vi "LVClass_ModalCoef ctor.vi"(0 "ModalCoef in":refnum<class "ModalCoef.lvclass">, 5 "TypePhase":T1, 11 "error in (no error)":errorcluster) -> (4 "ModalCoef out":refnum<class "ModalCoef.lvclass">, 15 "error out":errorcluster)   [LabVIEW 2020, in "ModalCoef.lvclass"]
doc: "ModalCoef constructor.\n\n--------------------------------------------------------------------------------\n\n<B>ModalCoefIn </B> : Constant Pointer to ModalCoef object.\n<B>ModalCoefOut </B> : Constant Pointer to ModalCoef object.\n<B>TypePhase </B> : TypePhase Phase mode reconstruction.\n<B>ErrorIn </B> : Error\n<B>ErrorOut </B> : Error\n\n--------------------------------------------------------------------------------"
uses:
  ModalCoef.lvclass
  WavefrontModalReconstructionType.ctl
  Handle creation.ctl
  ModalCoef.lvclass/ModalCoef.ctl
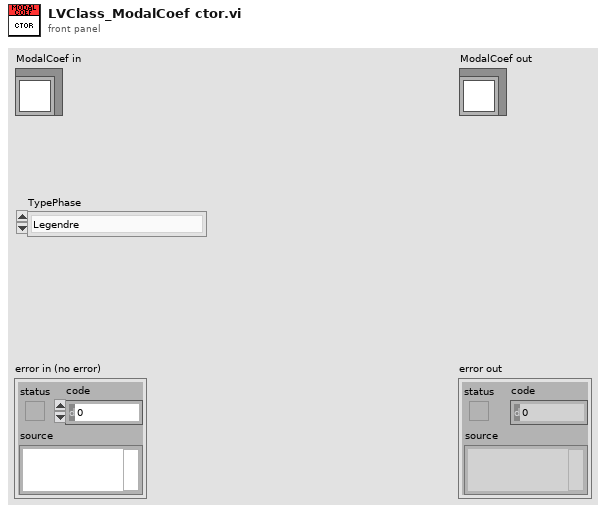
[diagram p1: front panel]
types:
  T1 = typedef "WavefrontModalReconstructionType.ctl" = enum16{"Legendre", "Zernike"}
  T2 = typedef "Handle creation.ctl" = enum16{"By ctor", "By write function"}
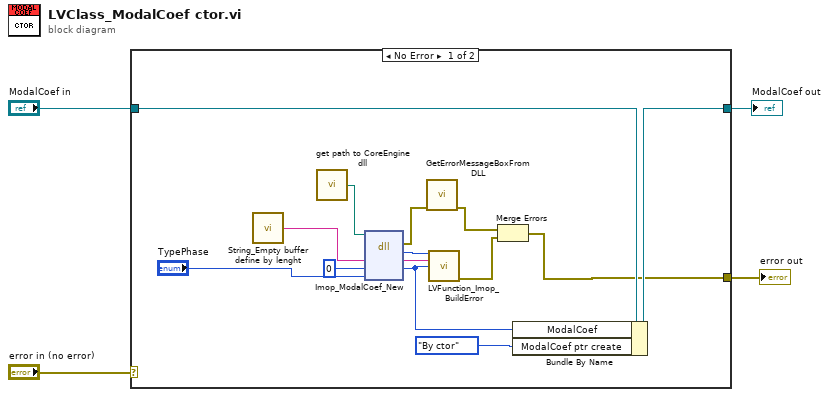
[diagram p0: block diagram]
diagram:
  n1 = case shown="No Error" "error in (no error)" {
    selector: "error in (no error)" -> [_ w20]
    tunnel: [w6 w20] -> w3
    tunnel: [w10 w19] -> w1
    tunnel: "ModalCoef in" -> [w11 w19]
    frame No Error {
      n2 = call "String_Empty buffer define by lenght.vi"() -> ("Empty buffer"=w18:string)  [unwired: 1 in]
      n3 = call "get path to CoreEngine dll.vi"() -> ("path to c_interface_vc100.dll"=w15:path)  [unwired: 12 in, 3 out]
      n4 = dll-call lib="D:/soft/HASO_v3/SVN_trunk/ImOpCoreEngine4_LV2011/DLLs/c_interface_vc100.dll" fn="Imop_ModalCoef_New"(path in=w15, "message"=w18, "ModalCoef"=0 ("Pupil"), "TypePhase"="TypePhase") -> (error out=w14:errorcluster, "return type"=w16:i32, "message"=w17:string, "ModalCoef"=w5:i32)  [unwired: 3 in, 1 out]
      n5 = call "GetErrorMessageBoxFromDLL.vi"("error IN"=w14) -> ("error OUT"=w8:errorcluster)  [unwired: 10 in]
      n6 = call "LVFunction_Imop_BuildError.vi"("code"=w16, "String to Prepend to source (\"\")"=w17, "Adresse"=w5) -> ("error out"=w7:errorcluster)  [unwired: 12 in]
      n7 = Merge Errors(w8, w7) -> (w6:errorcluster)
      n8 = Bundle By Name(cluster=w11, "ModalCoef"=w5, "ModalCoef ptr create"=Handle_creation."By ctor" ("Pupil ptr create")) -> (w10:refnum<class "ModalCoef.lvclass">)
    }
    frame Error {
    }
  }
  "error out" <- w3
  "ModalCoef out" <- w1
